vi "GOOP_GetLibWriterByLibRef.vi"(1 "Library Refnum":refnum<vi>, 5 "error in (no error)":errorcluster) -> (14 "LibWriter":refnum<class "LibWriter.lvclass">, 19 "error out":errorcluster)   [LabVIEW 2014]
uses:
  <resource>/Framework/Providers/Open_GDS/ClassProviders/LibProvider_BaseClassInterface/LibWriter_class/ClassWriter_class/LibWriter.lvclass
  <resource>/Framework/Providers/Open_GDS/ClassProviders/Provider_LvNativeClass/LvNativeProviderName.ctl
  <resource>/Framework/Providers/Open_GDS/ClassProviders/Provider_LvNativeClass/ClassWriterNative_class/ClassWriterNative.lvclass
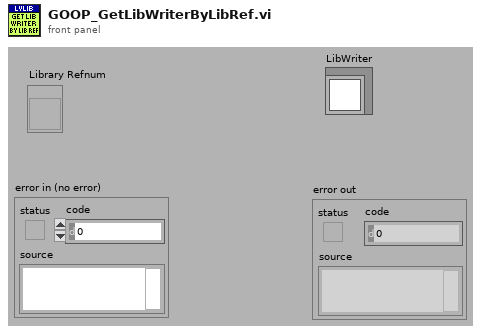
[diagram p1: front panel]
types:
  T1 = typedef "LvNativeProviderName.ctl" = enum16{"Endevo LabVIEW Native"}
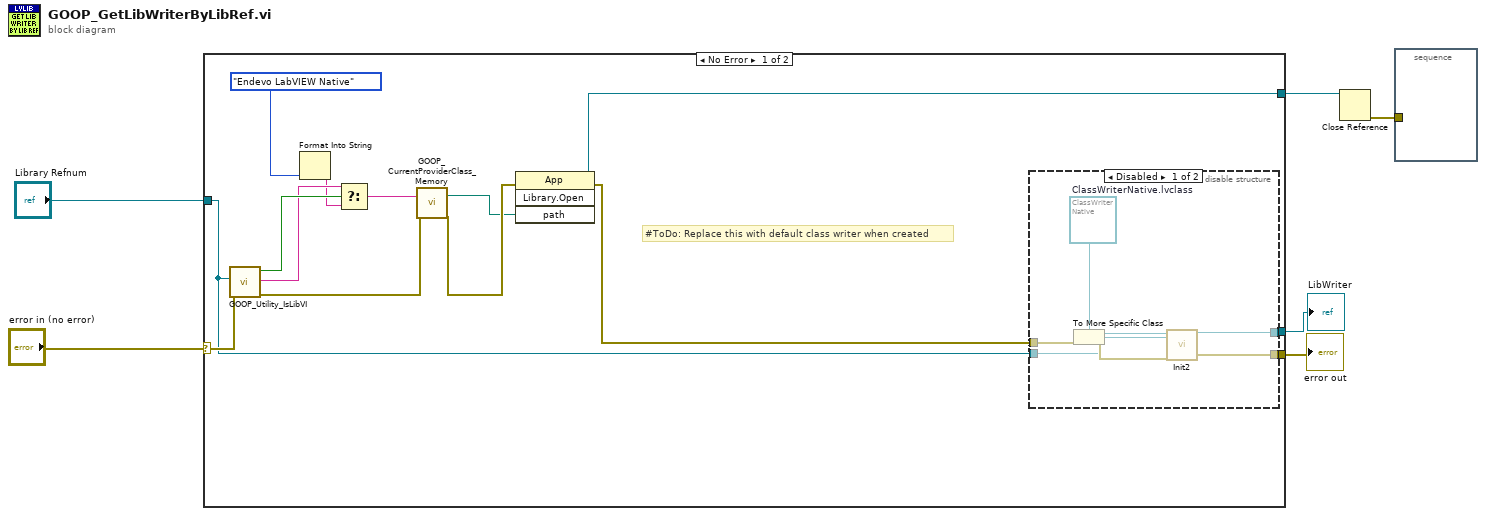
[diagram p0: block diagram]
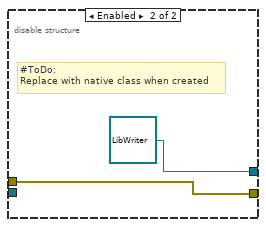
[diagram p2: hidden frame]
diagram:
  n1 = case shown="No Error" "error in (no error)" {
    selector: "error in (no error)" -> [w20 w30]
    tunnel: "Library Refnum" -> [w7 _]
    tunnel: [w11 w30] -> w4
    tunnel: [w12 _] -> w2
    tunnel: [w10 _] -> w3
    frame No Error {
      # "#ToDo: Replace this with default class writer when created"
      n2 = call <resource>:"GOOP_Utility_IsLibVI.vi"("error in (no error)"=w20, "ProjectItem"=w7) -> ("error out"=w19:errorcluster, "LibProvider"=w17:string, "Is Lib VI?"=w18:bool)  [unwired: 6 in, 1 out]
      n3 = Format Into String(LvNativeProviderName."Endevo LabVIEW Native" ("ProviderName")) -> (resulting string=w14:string)  [unwired: 3 in, 1 out]
      n4 = Select(t=w17, s=w18, f=w14) -> (s? t:f=w16:string)
      n5 = call <resource>:"GOOP_CurrentProviderClass_Memory.vi"("GetThisClassProvidersPaths(Returns the default providor if not wired)"=w16, "error in (no error)"=w19) -> ("ClassProviderClassWriterPath"=w8:path, "error out"=w13:errorcluster)  [unwired: 13 in, 3 out]
      n6 = invoke class="App" method="Library.Open"(error in=w13, "path"=w8) -> (reference out=w10:refnum<vi>, error out=w9:errorcluster)  [unwired: 2 in, 2 out]
      n7 = disable-structure shown="Disabled" {
        disable-tunnel: [w26 refnum<class "LibWriter.lvclass"> refnum ("LibWriter")] -> w12
        disable-tunnel: [w25 w28] -> w11
        disable-tunnel: w9 -> [w23 w28]
        disable-tunnel: w7 -> [w21 _]
        frame Disabled {
          w22 = refnum<class "ClassWriterNative.lvclass"> refnum  # ClassWriterNative.lvclass
          n8 = To More Specific Class(target class=w22, error in=w23) -> (specific class reference=w24:refnum<class "ClassWriterNative.lvclass">, error out=w27:errorcluster)  [unwired: 1 in]
          n9 = call-dynamic "Init2.vi"("ClassWriterNative.lvclass"=w24, "LvClassRef"=w21, "error in (no error)"=w27) -> ("ClassWriterNative.lvclass"=w26:refnum<class "ClassWriterNative.lvclass">, "error out"=w25:errorcluster)  [unwired: 15 in]
        }
        frame Enabled {
          # "#ToDo:\nReplace with native class when created"
        }
      }
    }
    frame Error {
    }
  }
  "error out" <- w4
  "LibWriter" <- w2
  n10 = Close Reference(reference=w3) -> (error out=w1:errorcluster)  [unwired: 1 in]
  n11 = stacked-sequence {
    tunnel: w1 -> [_]
    frame #0 {
    }
  }
